vi "ProgramReady(SubVI).vi"(8 "Error In":errorcluster, 11 "Boolean in":refnum<vi>) -> (0 "Error Out":errorcluster)   [LabVIEW 2018]
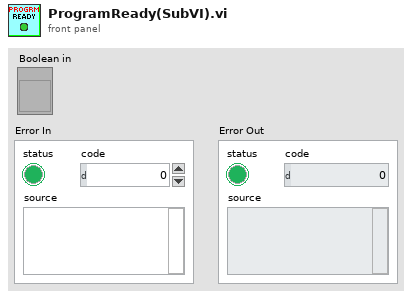
[diagram p1: front panel]
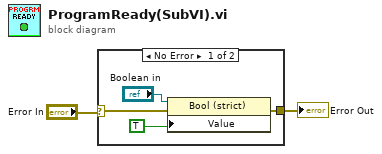
[diagram p0: block diagram]
diagram:
  n1 = case shown="No Error" "Error In" {
    selector: "Error In" -> [w4 w7]
    tunnel: [w3 w7] -> w1
    frame No Error {
      n2 = property on="Property Node" class="Bool (strict)"(reference="Boolean in", error in=w4, "Value"=TRUE ("Program busy")) -> (error out=w3:errorcluster)  [unwired: 1 out]
    }
    frame Error {
    }
  }
  "Error Out" <- w1
